vi "DT_Find Next Triangulation_Stop Check.vi"(9 "Data In":T1, 10 "Triangles In":i32[][](array[numeric]), 11 "Points In":cluster{"x":dbl, "y":dbl, "index":i32}[](array[cluster])) -> (0 "stop?":bool, 1 "Data Out":T1, 2 "Triangles Out":i32[][](array[numeric]), 3 "Points Out":cluster{"x":dbl, "y":dbl, "index":i32}[](array[cluster]))   [LabVIEW 2020, in "NI_AAL_Geometry.lvlib"]
uses:
  <vilib>/Analysis/NI_AAL_Geometry.lvlib
  <vilib>/Analysis/geometry.llb/DT_Find Next Triangulation_Data.ctl
  <vilib>/Analysis/geometry.llb/Triangle Area.vi
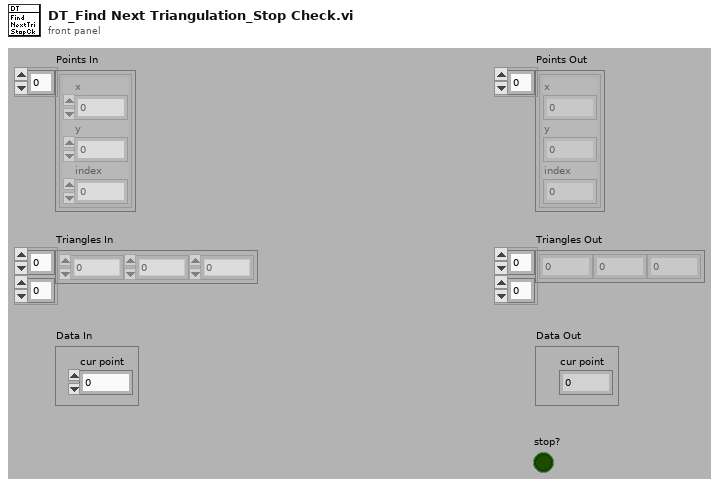
[diagram p1: front panel]
types:
  T1 = typedef "NI_AAL_Geometry.lvlib/DT_Find Next Triangulation_Data.ctl" = cluster{"cur point":i32, "cur triangle":i32, "cur local idx":i32, "base point":i32, "base triangle":i32, "base local idx":i32, "Candidate Triangles":i32[], "Candidate Point Idx":i32[]}
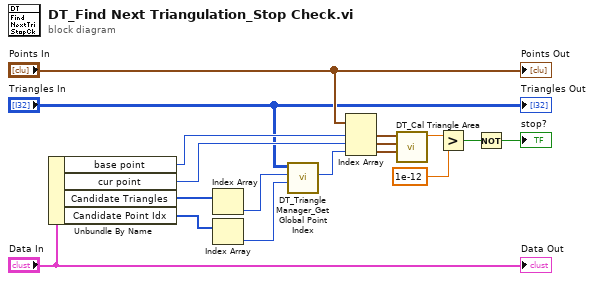
[diagram p0: block diagram]
diagram:
  n1 = Unbundle By Name("Data In") -> ("base point"=w9:i32, "cur point"=w8:i32, "Candidate Triangles"=w6:i32[], "Candidate Point Idx"=w5:i32[])
  n2 = Index Array(array=w6) -> (element=w4:i32)  [unwired: 1 in]
  n3 = Index Array(array=w5) -> (element=w3:i32)  [unwired: 1 in]
  n4 = call <vilib>:"DT_Triangle Manager_Get Global Point Index.vi"("local idx"=w3, "triangle"=w4, "Triangles"="Triangles In") -> ("global idx"=w2:i32)  [unwired: 8 out]
  n5 = Index Array(array="Points In", index #1=w9, index #2=w8, index #3=w2) -> (element #1=w14:cluster{"x":dbl, "y":dbl, "index":i32}, element #2=w13:cluster{"x":dbl, "y":dbl, "index":i32}, element #3=w12:cluster{"x":dbl, "y":dbl, "index":i32})
  n6 = call <vilib>:"DT_Cal Triangle Area.vi"("p 3"=w12, "p 2"=w13, "p 1"=w14) -> ("area"=w17:dbl)  [unwired: 8 out]
  n7 = Greater?(x=w17, y=1e-12 ("x")) -> (0:w11:bool)
  n8 = Not(x=w11) -> (.not. x?=→"stop?":bool)
  "Points Out" <- "Points In"
  "Triangles Out" <- "Triangles In"
  "Data Out" <- "Data In"
